vi "Facade.vi"(0 "Data In":T7, 2 "Display State In":T2={"WebView2 Ref"=refnum, "event callback refnum"=refnum, "Events"={"Navigation Complete Event"=refnum, "Source Changed Event"=refnum, "Document Title Changed Event"=refnum, "Status Bar Text Changed"=refnum, "Web Message Received"=refnum, "Window Close Requested"=refnum, "DOM Loaded"=refnum, "Navigation Started Event"=refnum}, "Paths"={"Webview2 Native"=path "C:/Users/kleins/Desktop/webview2/microsoft.web.webview2.1.0.1370.28/build/native", "Edge Application"=path "", "User Data"=path ""}, "Environment Options"={"additionalBrowserArguments"="", "language"="", "targetCompatibleBrowserVersion"="", "allowSingleSignOnUsingOSPrimaryAccount"=FALSE}}, 3 "Container State":T6) -> (6 "Data Out":T7, 7 "Display State Out":T2={"WebView2 Ref"=refnum, "event callback refnum"=refnum, "Events"={"Navigation Complete Event"=refnum, "Source Changed Event"=refnum, "Document Title Changed Event"=refnum, "Status Bar Text Changed"=refnum, "Web Message Received"=refnum, "Window Close Requested"=refnum, "DOM Loaded"=refnum, "Navigation Started Event"=refnum}, "Paths"={"Webview2 Native"=path "C:/Users/kleins/Desktop/webview2/microsoft.web.webview2.1.0.1370.28/build/native", "Edge Application"=path "", "User Data"=path ""}, "Environment Options"={"additionalBrowserArguments"="", "language"="", "targetCompatibleBrowserVersion"="", "allowSingleSignOnUsingOSPrimaryAccount"=FALSE}}, 8 "Action":T1)   [LabVIEW 2020, in "WebView2 Control.xctl"]
uses:
  WebView2 Control.xctl
  Data.ctl
  <vilib>/_xctls/Container State.ctl
  State.ctl
  E:/Labview/LV 2020/Libs/WebView2/LV-WebView2/Source/Libs/Microsoft.Web.WebView2.WinForms.dll
  Libs/Microsoft.Web.WebView2.WinForms.dll
  Events.ctl
  Paths.ctl
  Core Env Options.ctl
  <vilib>/_xctls/Action.ctl
  E:/Labview/LV 2020/Libs/WebView2/LV-WebView2/Source/Libs/Microsoft.Web.WebView2.Core.dll
  Libs/Microsoft.Web.WebView2.Core.dll
  <vilib>/_xctls/XControlSupport.lvlib
  Navigation Event Data.ctl
  Navigation Start Event Data.ctl
  Source Changed Event Data.ctl
panel:
  in  "WebView2":refnum<k24>(container)
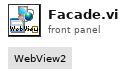
[diagram p1: front panel]
types:
  T1 = typedef "XControlSupport.lvlib/Action.ctl" = cluster{"Data Changed?":bool, "State Changed?":bool, "Action Name":string}
  T2 = typedef "WebView2 Control.xctl/State.ctl" = cluster{"WebView2 Ref":refnum<data-value>, "event callback refnum":refnum<k27>, "Events":T3, "Paths":T4, "Environment Options":T5}
  T3 = typedef "WebView2 Control.xctl/Events.ctl" = cluster{"Navigation Complete Event":refnum<user-event>, "Source Changed Event":refnum<user-event>, "Document Title Changed Event":refnum<user-event>, "Status Bar Text Changed":refnum<user-event>, "Web Message Received":refnum<user-event>, "Window Close Requested":refnum<user-event>, "DOM Loaded":refnum<user-event>, "Navigation Started Event":refnum<user-event>}
  T4 = typedef "WebView2 Control.xctl/Paths.ctl" = cluster{"Webview2 Native":path, "Edge Application":path, "User Data":path}
  T5 = typedef "WebView2 Control.xctl/Core Env Options.ctl" = cluster{"additionalBrowserArguments":string, "language":string, "targetCompatibleBrowserVersion":string, "allowSingleSignOnUsingOSPrimaryAccount":bool}
  T6 = typedef "XControlSupport.lvlib/Container State.ctl" = cluster{"Indicator?":bool, "Run Mode?":bool, " Refnum":refnum<vi>}
  T7 = typedef "WebView2 Control.xctl/Data.ctl" = string
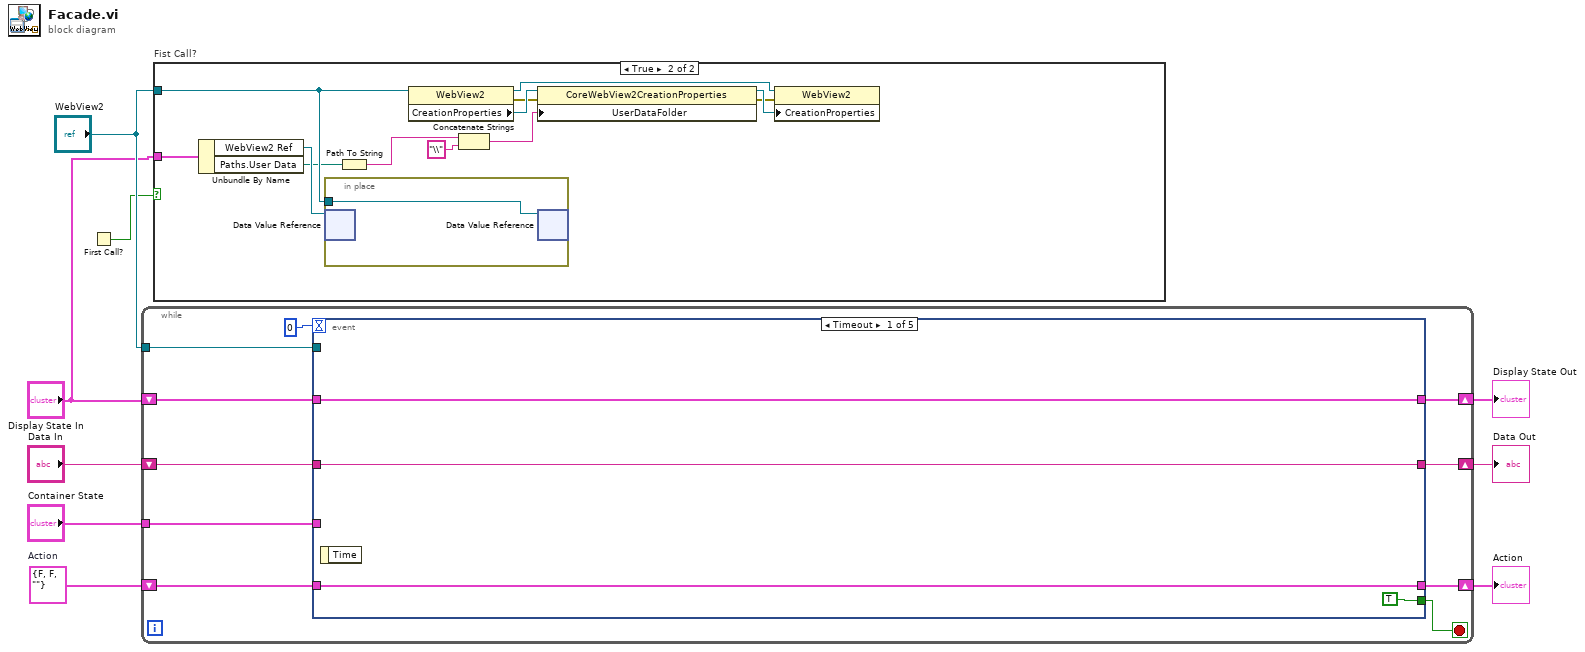
[diagram p0: block diagram]
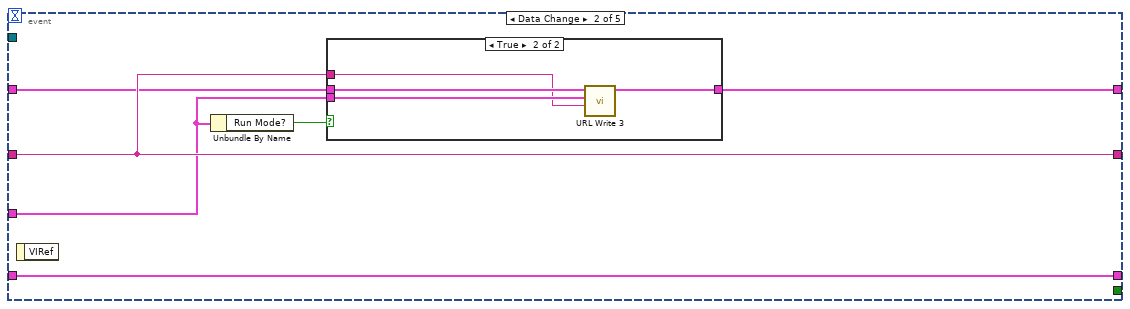
[diagram p2: hidden frame]
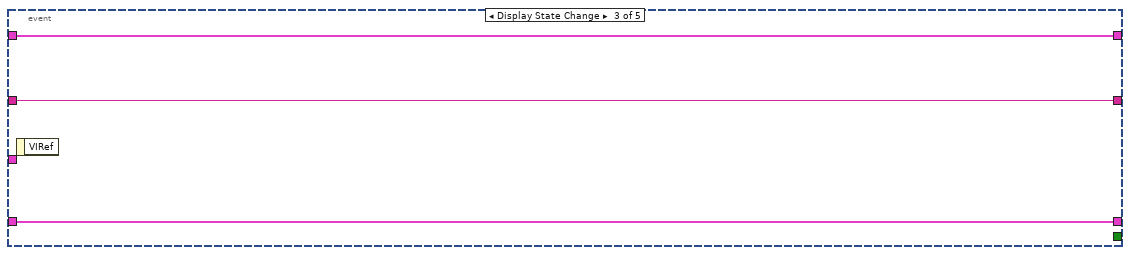
[diagram p4: hidden frame]
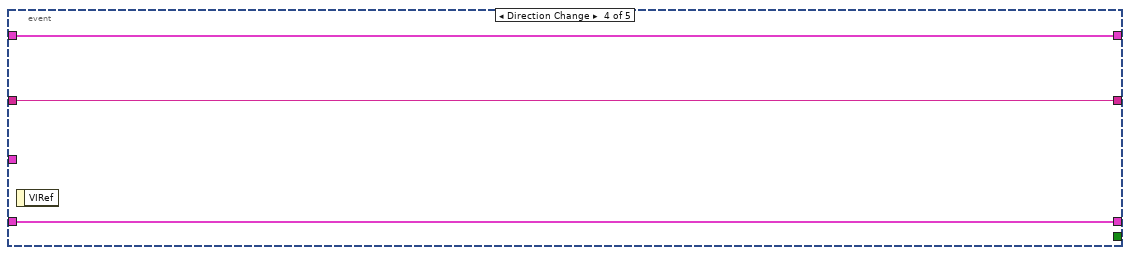
[diagram p5: hidden frame]
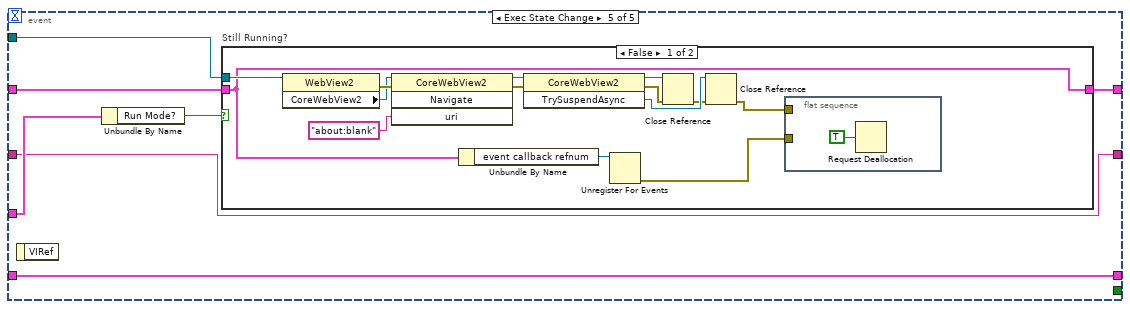
[diagram p6: hidden frame]
diagram:
  w5 = T1 {"Data Changed?"=FALSE, "State Changed?"=FALSE, "Action Name"=""}  # Action
  n1 = First Call?() -> (First Call?: T/F=w2:bool)
  n2 = while {
    tunnel: "WebView2" -> [w14]
    tunnel: "Container State" -> [w13]
    shift-right: [w19] -> w9
    shift-left: "Data In" -> [w18]
    shift-right: [w16] -> w6
    shift-left: w5 -> [w15]
    shift-right: [w17] -> w7
    shift-left: "Display State In" -> [w12]
    stop <- w10 stop-if-true
    n3 = event shown="[0] Timeout" {
      selector: _ -> [_ _ _ _ _]
      dyn-events: _ -> [_ _ _ _ _]
      timeout: 0 -> [_ _ _ _ _]
      tunnel: w12 -> [w21 w27 w37 w40 w42]
      tunnel: [w21 w24 w37 w40 w41] -> w17
      tunnel: [TRUE _ _ _ _] -> w10
      tunnel: w13 -> [_ w25 _ _ w47]
      tunnel: w18 -> [w20 w28 w36 w39 w46]
      tunnel: [w20 w28 w36 w39 w46] -> w19
      tunnel: [w22 w29 w35 w38 w45] -> w16
      tunnel: w15 -> [w22 w29 w35 w38 w45]
      tunnel: w14 -> [_ _ _ _ w44]
      event Timeout {
        n4 = event-data() -> ()  [unwired: 1 in, 1 out]
      }
      event Data Change {
        n5 = event-data() -> ()  [unwired: 1 in, 1 out]
        n6 = Unbundle By Name(w25) -> ("Run Mode?"=w26:bool)
        n7 = case shown="True" w26 {
          tunnel: w28 -> [_ w32]
          tunnel: w27 -> [w30 w34]
          tunnel: w25 -> [_ w33]
          tunnel: [w30 w31] -> w24
          frame False {
          }
          frame True {
            n8 = call "URL Write 3.vi"("Value"=w32, "Container State"=w33, "Display State In"=w34) -> ("Display State Out"=w31:T2)  [unwired: 3 in, 1 out]
          }
        }
      }
      event Display State Change {
        n9 = event-data() -> ()  [unwired: 1 in, 1 out]
      }
      event Direction Change {
        n10 = event-data() -> ()  [unwired: 1 in, 1 out]
      }
      event Exec State Change {
        n11 = event-data() -> ()  [unwired: 1 in, 1 out]
        n12 = Unbundle By Name(w47) -> ("Run Mode?"=w43:bool)
        n13 = case "Still Running?" shown="False" w43 {
          tunnel: w44 -> [w55 _]
          tunnel: w42 -> [w54 w63]
          tunnel: [w54 w63] -> w41
          frame False {
            n14 = property class="WebView2"(reference=w55) -> (error out=w60:errorcluster, "CoreWebView2"=w58:refnum<k24>)  [unwired: 1 in, 1 out]
            n15 = invoke class="CoreWebView2" method="Navigate"(reference=w58, error in=w60, "uri"="about:blank") -> (reference out=w57:refnum<k24>, error out=w59:errorcluster)  [unwired: 1 in, 2 out]
            n16 = Unbundle By Name(w54) -> ("event callback refnum"=w53:refnum<k27>)
            n17 = invoke class="CoreWebView2" method="TrySuspendAsync"(reference=w57, error in=w59) -> (reference out=w50:refnum<k24>, error out=w52:errorcluster, "TrySuspendAsync"=w61:refnum<k24>)  [unwired: 1 in]
            n18 = Unregister For Events(event registration refnum=w53) -> (error out=w48:errorcluster)  [unwired: 1 in]
            n19 = Close Reference(reference=w50, error in (no error)=w52) -> (error out=w51:errorcluster)
            n20 = Close Reference(reference=w61, error in (no error)=w51) -> (error out=w49:errorcluster)
            n21 = flat-sequence {
              tunnel: w49 -> [_]
              tunnel: w48 -> [_]
              frame #0 {
                n22 = Request Deallocation(TRUE ("flag")) -> ()
              }
            }
          }
          frame True {
          }
        }
      }
    }
  }
  "Display State Out" <- w7
  "Data Out" <- w9
  "Action" <- w6
  n23 = case "Fist Call?" shown="True" w2 {
    tunnel: "WebView2" -> [_ w71]
    tunnel: "Display State In" -> [_ w69]
    frame False {
    }
    frame True {
      n24 = Unbundle By Name(w69) -> ("WebView2 Ref"=w68:refnum<data-value>, "Paths.User Data"=w67:path)
      n25 = in-place {
        in-place-border: w71 -> [w76]
        n26 = in-place-dvr #1(w68) -> ()  [unwired: 2 out]
        n27 = in-place-dvr #1(w76) -> ()  [unwired: 2 out]
      }
      n28 = Path To String(path=w67) -> (string=w66:string)
      n29 = property class="WebView2"(reference=w71) -> (reference out=w70:refnum<k24>, error out=w72:errorcluster, "CreationProperties"=w75:refnum<k24>)  [unwired: 1 in]
      n30 = Concatenate Strings(w66, "\\" ("string")) -> (w64:string)
      n31 = property class="CoreWebView2CreationProperties"(reference=w75, error in=w72, "UserDataFolder"=w64) -> (reference out=w74:refnum<k24>, error out=w73:errorcluster)
      n32 = property class="WebView2"(reference=w70, error in=w73, "CreationProperties"=w74) -> ()  [unwired: 2 out]
    }
  }
